vi "HEUI.vi"(0 "LED Update Rate (s)":dbl=0.25 caption="Delay Time (s)", 6 "HEUI_Buttons":T1={"SW204 - Signal Adjust"=FALSE, "SW203 - Extra Rinse"=FALSE, "SW201 - My Cycle"=FALSE, "SW202 - Delay Wash"=FALSE, "SW211 - Deep Fill"=FALSE, "SW210 - Warm Rinse"=FALSE, "SW208 - Auto Soak"=FALSE, "SW206 - Deep Rinse"=FALSE, "SW209 - Temp"=FALSE, "SW207 - Soil"=FALSE, "SW205 - Spin"=FALSE, "SW212 - Stains"=FALSE, "Cycle Selection"=enum."Cycle 0", "SW213 - Power"=FALSE, "SW214 - Start/Pause"=FALSE}, 7 "stop":bool, 11 "Error In":errorcluster) -> (5 "HEUI_LEDs":T2, 15 "Error Out":errorcluster)   [LabVIEW 2016]
doc: "This VI controls the high end 2015 VA washer UI board. The VI updates the status of the LEDs every 'LED update rate (s)' number of seconds. The VI allows the user to press buttons and select a cycle."
uses:
  Laundry Tool Support/type defs/HEUI_Buttons.ctl
  Automation/Product Specific/Clothes Care/TL27/Product Testcode/VALEW/Valew Common/Display/controls/HEUI_LEDs.ctl
  Common/LabVIEW GEA2 Toolkit/LabVIEW_GEA2_Toolkit.lvlibp/type defs/Data In.ctl
  Common/LabVIEW GEA2 Toolkit/LabVIEW_GEA2_Toolkit.lvlibp/type defs/Source_Destination.ctl
  Common/LabVIEW GEA2 Toolkit/LabVIEW_GEA2_Toolkit.lvlibp/type defs/ERD Read Data In.ctl
  Common/LabVIEW GEA2 Toolkit/LabVIEW_GEA2_Toolkit.lvlibp/type defs/Data Type.ctl
  Common/LabVIEW GEA2 Toolkit/LabVIEW_GEA2_Toolkit.lvlibp/type defs/ERD Write Data In.ctl
  Automation/Product Specific/Clothes Care/TL27/Product Testcode/VALEW/Valew Common/type defs/UI Buttons.ctl
  Common/LabVIEW GEA2 Toolkit/LabVIEW_GEA2_Toolkit.lvlibp
  Automation/Product Specific/Clothes Care/TL27/Projects/TL27.lvlib
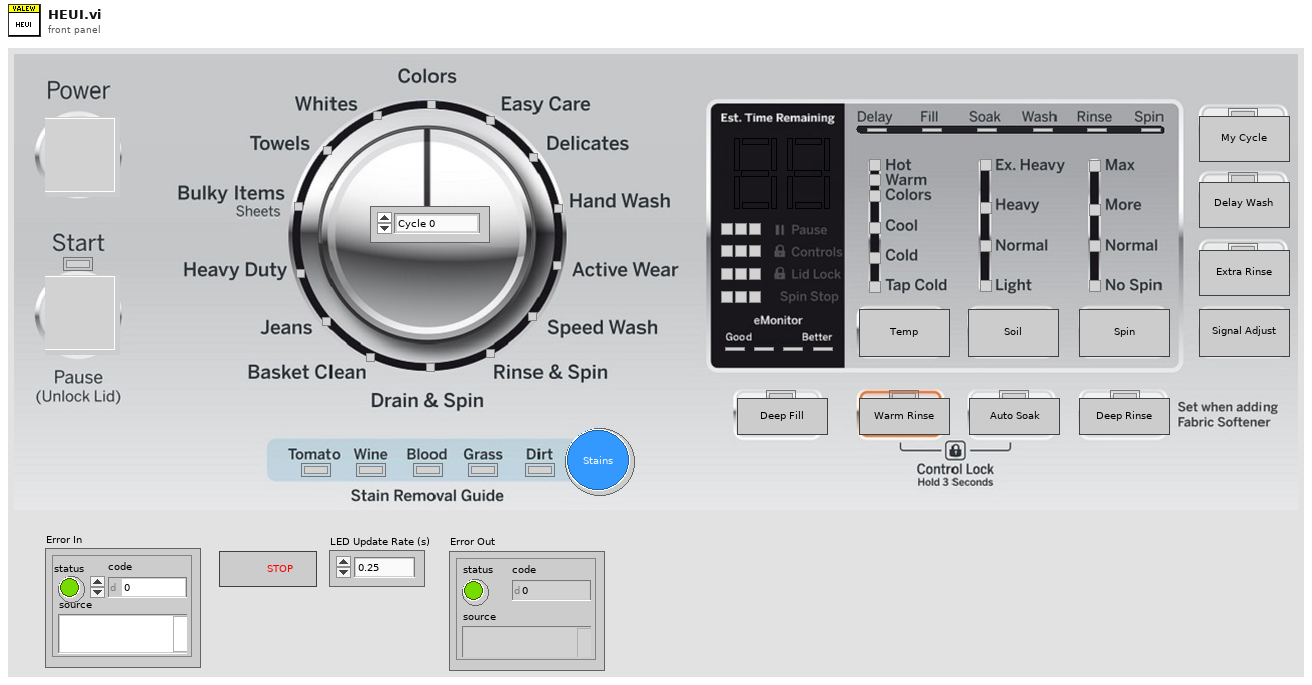
[diagram p1: front panel]
types:
  T1 = typedef "HEUI_Buttons.ctl" = cluster{"SW204 - Signal Adjust":bool, "SW203 - Extra Rinse":bool, "SW201 - My Cycle":bool, "SW202 - Delay Wash":bool, "SW211 - Deep Fill":bool, "SW210 - Warm Rinse":bool, "SW208 - Auto Soak":bool, "SW206 - Deep Rinse":bool, "SW209 - Temp":bool, "SW207 - Soil":bool, "SW205 - Spin":bool, "SW212 - Stains":bool, "Cycle Selection":enum16{"Cycle 13", "Cycle 12", "Cycle 11", "Cycle 10", "Cycle 9", "Cycle 8", "Cycle 7", "Cycle 6", "Cycle 5", "Cycle 4", "Cycle 3", "Cycle 2", "Cycle 1", "Cycle 0"}, "SW213 - Power":bool, "SW214 - Start/Pause":bool}
  T2 = typedef "TL27.lvlib/HEUI_LEDs.ctl" = cluster{"Z101 - Start":bool, "Z103 - Colors":bool, "Z104 - Whites":bool, "Z105 - Towels":bool, "Z106 - Bulky Items":bool, "Z107 - Heavy Duty":bool, "Z108 - Jeans":bool, "Z109 - Basket Clean":bool, "Z110 - Drain and Spin":bool, "Z111 - Rinse and Spin":bool, "Z112 - Speed Wash":bool, "Z113 - Active Wear":bool, "Z114 - Hand Wash":bool, "Z115 - Delicates":bool, "Z116 - Easy Care":bool, "Z117 - Tomato":bool, "Z118 - Wine":bool, "Z119 - Blood":bool, "Z120 - Grass":bool, "Z121 - Dirt":bool, "Z122_MSB_A":bool, "Z123_MSB_B":bool, "Z124_MSB_G":bool, "Z125_MSB_C":bool, "Z126_MSB_D":bool, "Z127_MSB_E":bool, "Z128_MSB_F":bool, "Z129_LSB_A":bool, "Z130_LSB_B":bool, "Z131_LSB_G":bool, "Z132_LSB_C":bool, "Z133_LSB_D":bool, "Z134_LSB_E":bool, "Z135_LSB_F":bool, "Z136 - Pause":bool, "Z137 - Pause":bool, "Z138 - Lock Controls":bool, "Z139 - Lock Controls":bool, "Z140 - Lock Controls":bool, "Z141 - Lid Lock":bool, "Z142 - Lid Lock":bool, "Z143 - Lid Lock":bool, "Z144 - Good":bool, "Z145":bool, "Z146":bool, "Z147 - Better":bool, "Z148 - Delay":bool, "Z149 - Fill":bool, "Z150 - Soak":bool, "Z151 - Wash":bool, "Z152 - Rinse":bool, "Z153 - Spin":bool, "Z154 - Hot":bool, "Z155 - Warm":bool, "Z156 - Colors":bool, "Z157 - Cool":bool, "Z158 - Cold":bool, "Z159 - Tap Cold":bool, "Z160 - Extra Heavy":bool, "Z161 - Heavy":bool, "Z162 - Normal":bool, "Z163 - Light":bool, "Z164 - Max Spin":bool, "Z165 - More Spin":bool, "Z166 - Normal Spin":bool, "Z167 - No Spin":bool, "Z168 - Extra Rinse":bool, "Z170 - Deep Rinse":bool, "Z171 - Auto Soak":bool, "Z172 - Warm Rinse":bool, "Z173 - Deep Fill":bool, "Z174 - My Cycles":bool, "Z175 - Delay Wash":bool, "Z176 - Spin Stop":bool, "Z177 - Spin Stop":bool, "Z178 - Spin Stop":bool, "Z179 - Pause":bool, "Z109":bool, "Z110":bool, "Z123":bool, "Z124":bool, "Z140":bool, "Unused0":bool, "Unused1":bool, "Unused2":bool, "Unused3":bool, "Channel_Off":bool, "Channel_Cycle_Unmapped":bool}
  T3 = typedef "LabVIEW_GEA2_Toolkit.lvlibp/ERD Write Data In.ctl" = cluster{"ERD Number":u16, "Data Type":T4, "Data":string}
  T4 = typedef "LabVIEW_GEA2_Toolkit.lvlibp/Data Type.ctl" = enum16{"string", "boolean", "uint8_t", "uint16_t", "uint32_t", "uint64_t", "int8_t", "int16_t", "int32_t", "int64_t"}
  T5 = typedef "LabVIEW_GEA2_Toolkit.lvlibp/ERD Read Data In.ctl" = cluster{"ERD Number":u16, "Data Type":T4}
  T6 = typedef "LabVIEW_GEA2_Toolkit.lvlibp/Source_Destination.ctl" = cluster{"Source":u8, "Destination":u8}
  T7 = typedef "LabVIEW_GEA2_Toolkit.lvlibp/Data In.ctl" = cluster{"Source":u8, "Destination":u8, "Command":u8, "Message":string}
  T8 = typedef "TL27.lvlib/UI Buttons.ctl" = enum16{"Switch Off", "SW201 - My Cycle", "SW202 - Delay Wash", "SW203 - Extra Rinse", "SW204 - Signal / Volume", "SW205 - Spin", "SW206 - Deep Rinse / Fab Soft", "SW207 - Soil", "SW208 - Auto Soak", "SW209 - Temp", "SW210 - Warm Rinse", "SW211 - Deep Fill", "SW212 - Stain Remover", "SW213 - Power", "SW222 - Control Lock", "SW214 - Start / Pause", "SW301 - Start/Pause LE", "SW302 - Option Button LE", "SW201/212 - Bulk Flush"}
  T9 = enum16{"string", "boolean", "uint8_t", "uint16_t", "uint32_t"}
  T10 = enum16{"Cycle 13", "Cycle 12", "Cycle 11", "Cycle 10", "Cycle 9", "Cycle 8", "Cycle 7", "Cycle 6", "Cycle 5", "Cycle 4", "Cycle 3", "Cycle 2", "Cycle 1", "Cycle 0"}
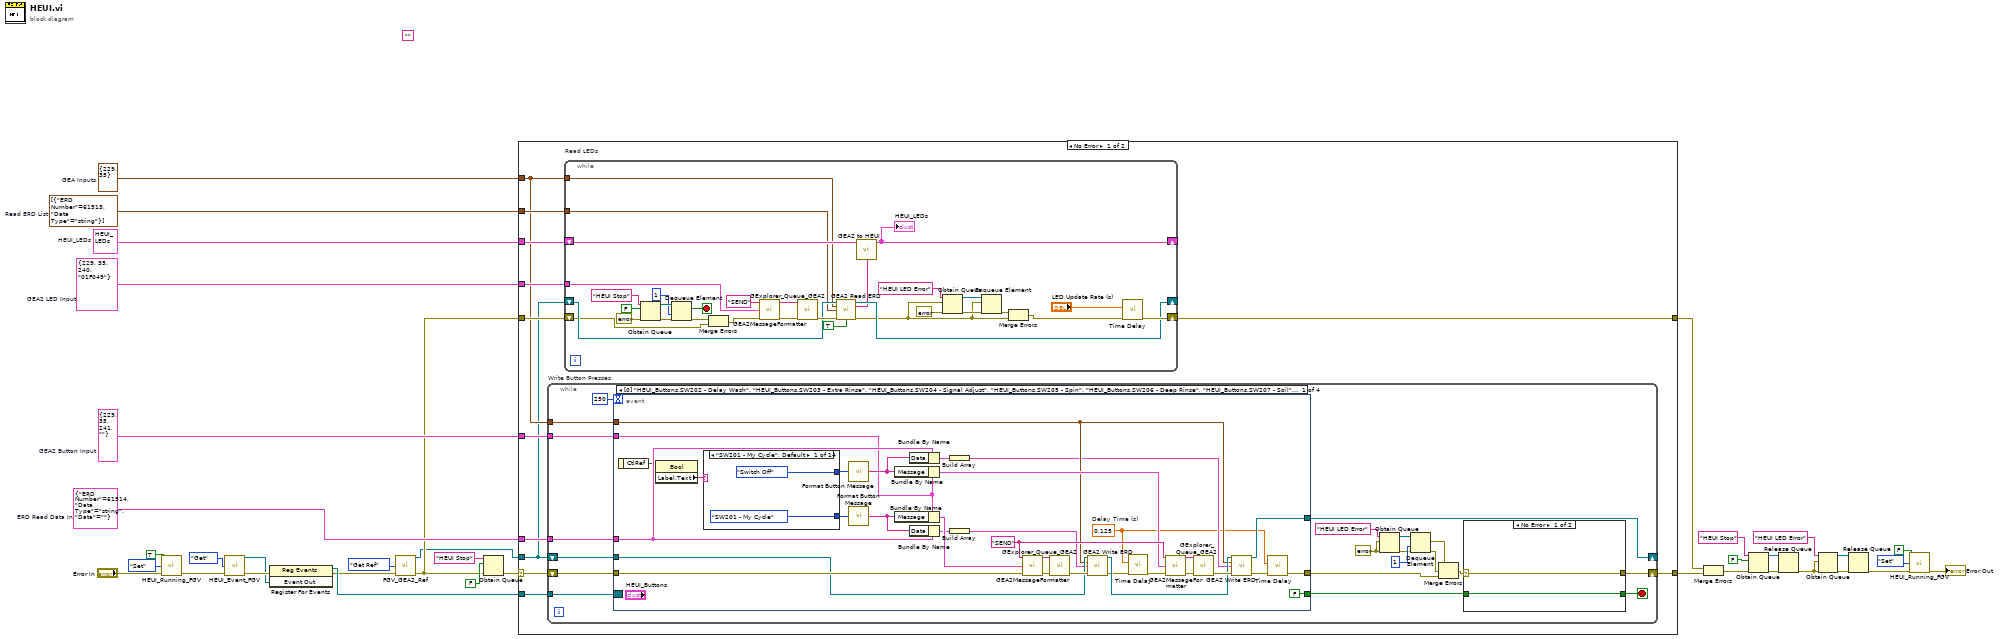
[diagram p0: block diagram]
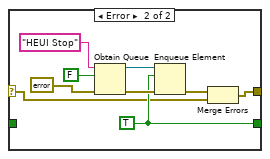
[diagram p2: hidden frame]
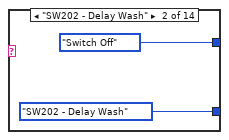
[diagram p3: hidden frame]
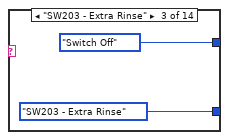
[diagram p4: hidden frame]
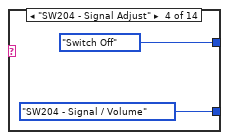
[diagram p5: hidden frame]
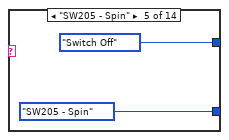
[diagram p6: hidden frame]
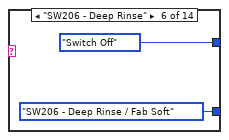
[diagram p7: hidden frame]
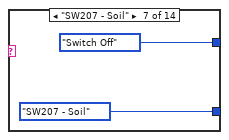
[diagram p8: hidden frame]
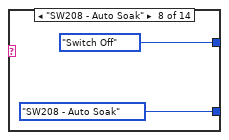
[diagram p9: hidden frame]
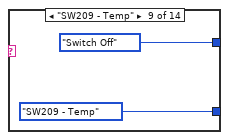
[diagram p10: hidden frame]
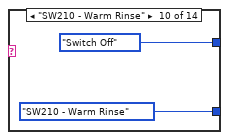
[diagram p11: hidden frame]
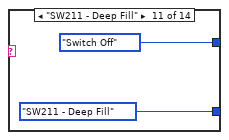
[diagram p12: hidden frame]
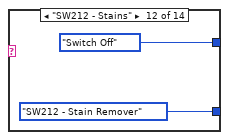
[diagram p13: hidden frame]
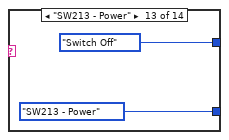
[diagram p14: hidden frame]
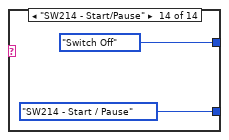
[diagram p15: hidden frame]
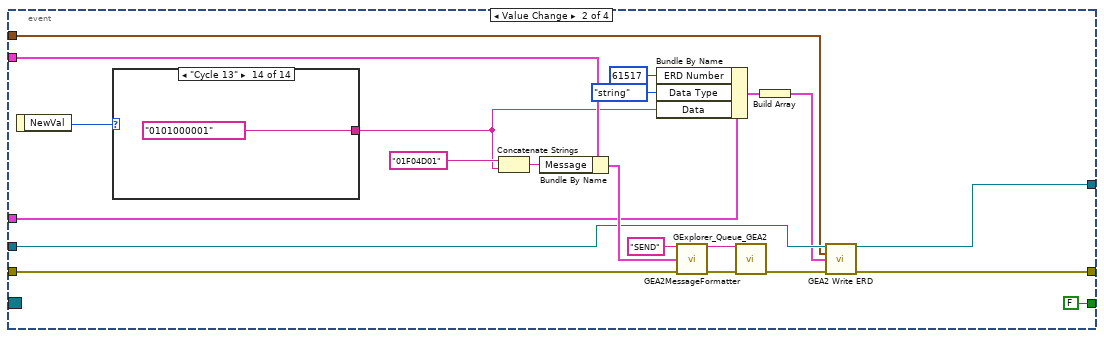
[diagram p16: hidden frame]
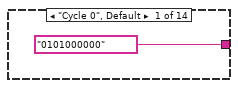
[diagram p17: hidden frame]
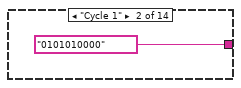
[diagram p18: hidden frame]
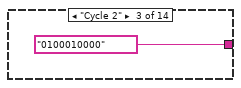
[diagram p19: hidden frame]
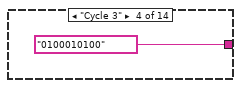
[diagram p20: hidden frame]
diagram:
  w24 = T3 {"ERD Number"=61514, "Data Type"=enum."string", "Data"=""}  # ERD Read Data In
  w26 = T5[] [{"ERD Number"=61513, "Data Type"=enum."string"}]  # Read ERD List
  w25 = T6 {"Source"=229, "Destination"=35}  # GEA Inputs
  w34 = T7 {"Source"=229, "Destination"=35, "Command"=240, "Message"="01F049"}  # GEA2 LED Input
  w35 = T2 {"Z101 - Start"=FALSE, "Z103 - Colors"=FALSE, "Z104 - Whites"=FALSE, "Z105 - Towels"=FALSE, "Z106 - Bulky Items"=FALSE, "Z107 - Heavy Duty"=FALSE, "Z108 - Jeans"=FALSE, "Z109 - Basket Clean"=FALSE, "Z110 - Drain and Spin"=FALSE, "Z111 - Rinse and Spin"=FALSE, "Z112 - Speed Wash"=FALSE, "Z113 - Active Wear"=FALSE, "Z114 - Hand Wash"=FALSE, "Z115 - Delicates"=FALSE, "Z116 - Easy Care"=FALSE, "Z117 - Tomato"=FALSE, "Z118 - Wine"=FALSE, "Z119 - Blood"=FALSE, "Z120 - Grass"=FALSE, "Z121 - Dirt"=FALSE, "Z122_MSB_A"=FALSE, "Z123_MSB_B"=FALSE, "Z124_MSB_G"=FALSE, "Z125_MSB_C"=FALSE, "Z126_MSB_D"=FALSE, "Z127_MSB_E"=FALSE, "Z128_MSB_F"=FALSE, "Z129_LSB_A"=FALSE, "Z130_LSB_B"=FALSE, "Z131_LSB_G"=FALSE, "Z132_LSB_C"=FALSE, "Z133_LSB_D"=FALSE, "Z134_LSB_E"=FALSE, "Z135_LSB_F"=FALSE, "Z136 - Pause"=FALSE, "Z137 - Pause"=FALSE, "Z138 - Lock Controls"=FALSE, "Z139 - Lock Controls"=FALSE, "Z140 - Lock Controls"=FALSE, "Z141 - Lid Lock"=FALSE, "Z142 - Lid Lock"=FALSE, "Z143 - Lid Lock"=FALSE, "Z144 - Good"=FALSE, "Z145"=FALSE, "Z146"=FALSE, "Z147 - Better"=FALSE, "Z148 - Delay"=FALSE, "Z149 - Fill"=FALSE, "Z150 - Soak"=FALSE, "Z151 - Wash"=FALSE, "Z152 - Rinse"=FALSE, "Z153 - Spin"=FALSE, "Z154 - Hot"=FALSE, "Z155 - Warm"=FALSE, "Z156 - Colors"=FALSE, "Z157 - Cool"=FALSE, "Z158 - Cold"=FALSE, "Z159 - Tap Cold"=FALSE, "Z160 - Extra Heavy"=FALSE, "Z161 - Heavy"=FALSE, "Z162 - Normal"=FALSE, "Z163 - Light"=FALSE, "Z164 - Max Spin"=FALSE, "Z165 - More Spin"=FALSE, "Z166 - Normal Spin"=FALSE, "Z167 - No Spin"=FALSE, "Z168 - Extra Rinse"=FALSE, "Z170 - Deep Rinse"=FALSE, "Z171 - Auto Soak"=FALSE, "Z172 - Warm Rinse"=FALSE, "Z173 - Deep Fill"=FALSE, "Z174 - My Cycles"=FALSE, "Z175 - Delay Wash"=FALSE, "Z176 - Spin Stop"=FALSE, "Z177 - Spin Stop"=FALSE, "Z178 - Spin Stop"=FALSE, "Z179 - Pause"=FALSE, "Z109"=FALSE, "Z110"=FALSE, "Z123"=FALSE, "Z124"=FALSE, "Z140"=FALSE, "Unused0"=FALSE, "Unused1"=FALSE, "Unused2"=FALSE, "Unused3"=FALSE, "Channel_Off"=FALSE, "Channel_Cycle_Unmapped"=FALSE}  # HEUI_LEDs
  w33 = T7 {"Source"=229, "Destination"=35, "Command"=241, "Message"=""}  # GEA2 Button Input
  (unwired) ""
  n1 = call "HEUI_Running_FGV.vi"("Running?"=TRUE, "Action"=enum16{"Get", "Set"}."Set", "Error In"="Error In") -> ("Error Out"=w8:errorcluster)  [unwired: 11 in, 1 out]
  n2 = call "HEUI_Event_FGV.vi"("Action"=enum16{"Get", "Set"}."Get", "Error In"=w8) -> ("Event Out"=w15:refnum<user-event>, "Error Out"=w16:errorcluster)  [unwired: 12 in]
  n3 = register-events(error in=w16, w15) -> (reference out=w18:refnum<event-registration>, error out=w12:errorcluster)  [unwired: 1 in]
  n4 = call "FGV_GEA2_Ref.vi"("Action"=enum16{"Set Ref", "Get Ref"}."Get Ref", "Error In"=w12) -> ("GEA2 Reference Out"=w10:refnum<k24>, "Error Out"=w11:errorcluster)  [unwired: 12 in]
  n5 = Obtain Queue(name (unnamed)="HEUI Stop", element data type=FALSE ("stop"), error in (no error)=w11) -> (error out=w23:errorcluster)  [unwired: 2 in, 2 out]
  n6 = case shown="No Error" w23 {
    selector: w23 -> [w38 w238]
    tunnel: w10 -> [w39 _]
    tunnel: [w48 errorcluster {"status"=FALSE, "code"=0, "source"=""} ("error out")] -> w36
    tunnel: [w47 w238] -> w9
    tunnel: w35 -> [w46 _]
    tunnel: w34 -> [w45 _]
    tunnel: w33 -> [w44 _]
    tunnel: w11 -> [w43 _]
    tunnel: w26 -> [w42 _]
    tunnel: w25 -> [w41 _]
    tunnel: w24 -> [w40 _]
    tunnel: w18 -> [w37 _]
    frame No Error {
      n7 = while "Write Button Presses" {
        shift-right: [w94] -> w47
        shift-left: w38 -> [w100]
        shift-right: [w98] -> _
        shift-left: w39 -> [w99]
        tunnel: w44 -> [w97]
        tunnel: w41 -> [w96]
        tunnel: w40 -> [w95]
        tunnel: w37 -> [w81]
        stop <- w92 stop-if-true
        w86 = errorcluster {"status"=FALSE, "code"=0, "source"=""} ("error in (no error)")
        n8 = event shown="[0] \"HEUI_Buttons.SW202 - Delay Wash\", \"HEUI_Buttons.SW203 - Extra Rinse\", \"HEUI_Buttons.SW204 - Signal Adjust\", \"HEUI_Buttons.SW205 - Spin\", \"HEUI_Buttons.SW206 - Deep Rinse\", \"HEUI_Buttons.SW207 - Soil\", \"HEUI_Buttons.SW208 - Auto Soak\", \"HEUI_Buttons.SW209 - Temp\", \"HEUI_Buttons.SW210 - Warm Rinse\", \"HEUI_Buttons.SW211 - Deep Fill\", \"HEUI_Buttons.SW212 - Stains\", \"HEUI_Buttons.SW213 - Power\", \"HEUI_Buttons.SW214 - Start/Pause\", \"HEUI_Buttons.SW201 - My Cycle\": Value Change" {
          selector: w81 -> [_ _ _ _]
          dyn-events: _ -> [_ _ _ _]
          timeout: 250 -> [_ _ _ _]
          tunnel: [w120 w184 w232 w235] -> w84
          tunnel: w100 -> [w142 w192 w213 w235]
          tunnel: w99 -> [w134 w183 w209 w236]
          tunnel: [w132 w182 w207 w236] -> w98
          tunnel: [FALSE ("stop") FALSE ("stop") w231 FALSE ("stop")] -> w93
          tunnel: w97 -> [w117 w191 w215 _]
          tunnel: w96 -> [w130 w181 w208 _]
          tunnel: w95 -> [w125 w180 w211 _]
          event Value Change {
            w116 = 0.125  # Delay Time (s)
            w140 = "SEND" ("Prefix(Send/Recv)")
            n9 = event-data() -> ("CtlRef"=w119:refnum<vi>)  [unwired: 1 in]
            n10 = property class="Bool"(reference=w119) -> ("Label.Text"=w118:string)  [unwired: 1 in, 2 out]
            n11 = case shown="\"SW201 - My Cycle\", Default" w118 {
              tunnel: [UI_Buttons."SW201 - My Cycle" ("Switch") UI_Buttons."SW202 - Delay Wash" ("Switch") UI_Buttons."SW203 - Extra Rinse" ("Switch") UI_Buttons."SW204 - Signal / Volume" ("Switch") UI_Buttons."SW205 - Spin" ("Switch") UI_Buttons."SW206 - Deep Rinse / Fab Soft" ("Switch") UI_Buttons."SW207 - Soil" ("Switch") UI_Buttons."SW208 - Auto Soak" ("Switch") UI_Buttons."SW209 - Temp" ("Switch") UI_Buttons."SW210 - Warm Rinse" ("Switch") UI_Buttons."SW211 - Deep Fill" ("Switch") UI_Buttons."SW212 - Stain Remover" ("Switch") UI_Buttons."SW213 - Power" ("Switch") UI_Buttons."SW214 - Start / Pause" ("Switch")] -> w113
              tunnel: [UI_Buttons."Switch Off" ("Switch") UI_Buttons."Switch Off" ("Switch") UI_Buttons."Switch Off" ("Switch") UI_Buttons."Switch Off" ("Switch") UI_Buttons."Switch Off" ("Switch") UI_Buttons."Switch Off" ("Switch") UI_Buttons."Switch Off" ("Switch") UI_Buttons."Switch Off" ("Switch") UI_Buttons."Switch Off" ("Switch") UI_Buttons."Switch Off" ("Switch") UI_Buttons."Switch Off" ("Switch") UI_Buttons."Switch Off" ("Switch") UI_Buttons."Switch Off" ("Switch") UI_Buttons."Switch Off" ("Switch")] -> w114
              frame "SW201 - My Cycle", Default {
              }
              frame "SW202 - Delay Wash" {
              }
              frame "SW203 - Extra Rinse" {
              }
              frame "SW204 - Signal Adjust" {
              }
              frame "SW205 - Spin" {
              }
              frame "SW206 - Deep Rinse" {
              }
              frame "SW207 - Soil" {
              }
              frame "SW208 - Auto Soak" {
              }
              frame "SW209 - Temp" {
              }
              frame "SW210 - Warm Rinse" {
              }
              frame "SW211 - Deep Fill" {
              }
              frame "SW212 - Stains" {
              }
              frame "SW213 - Power" {
              }
              frame "SW214 - Start/Pause" {
              }
            }
            n12 = call "Format Button Message.vi"("Switch"=w114) -> ("Switch Message"=w129:string)  [unwired: 14 in]
            n13 = call "Format Button Message.vi"("Switch"=w113) -> ("Switch Message"=w112:string)  [unwired: 14 in]
            n14 = Bundle By Name(cluster=w117, "Message"=w129) -> (w136:T7)
            n15 = Bundle By Name(cluster=w117, "Message"=w112) -> (w137:T7)
            n16 = Bundle By Name(cluster=w125, "Data"=w129) -> (w128:T3)
            n17 = Bundle By Name(cluster=w125, "Data"=w112) -> (w126:T3)
            n18 = Build Array(w128) -> (w127:T3[])
            n19 = Build Array(w126) -> (w124:T3[])
            n20 = call "GEA2MessageFormatter.vi"("Prefix(Send/Recv)"=w140, "GEA2 Data In"=w137, "Error In"=w142) -> ("Output String"=w139:string, "Error Out"=w143:errorcluster)  [unwired: 11 in]
            n21 = call "GExplorer_Queue_GEA2.vi"("Output String"=w139, "error in (no error)"=w143) -> ("error out"=w135:errorcluster)  [unwired: 13 in]
            n22 = call "GEA2 Write ERD.vi"("GEA2 Reference In"=w134, "GEA Inputs"=w130, "Write ERD List"=w124, "Error In"=w135) -> ("GEA2 Reference Out"=w131:refnum<k24>, "Error Out"=w123:errorcluster)  [unwired: 9 in, 1 out]
            n23 = call "Time Delay"("error in (no error)"=w123, "Delay Time (s)"=w116) -> ("error out"=w122:errorcluster)  [unwired: 9 in]
            n24 = call "GEA2MessageFormatter.vi"("Prefix(Send/Recv)"=w140, "GEA2 Data In"=w136, "Error In"=w122) -> ("Output String"=w138:string, "Error Out"=w141:errorcluster)  [unwired: 11 in]
            n25 = call "GExplorer_Queue_GEA2.vi"("Output String"=w138, "error in (no error)"=w141) -> ("error out"=w133:errorcluster)  [unwired: 13 in]
            n26 = call "GEA2 Write ERD.vi"("GEA2 Reference In"=w131, "GEA Inputs"=w130, "Write ERD List"=w127, "Error In"=w133) -> ("GEA2 Reference Out"=w132:refnum<k24>, "Error Out"=w121:errorcluster)  [unwired: 9 in, 1 out]
            n27 = call "Time Delay"("error in (no error)"=w121, "Delay Time (s)"=w116) -> ("error out"=w120:errorcluster)  [unwired: 9 in]
          }
          event Value Change {
            n28 = event-data() -> ("NewVal"=w175:T10)  [unwired: 1 in]
            n29 = case shown="\"Cycle 13\"" w175 {
              tunnel: ["0101000000" "0101010000" "0100010000" "0100010100" "0101010100" "0101000100" "0100000100" "0100000101" "0101000101" "0101010101" "0100010101" "0100010001" "0101010001" "0101000001"] -> w173
              frame "Cycle 0", Default {
              }
              frame "Cycle 1" {
              }
              frame "Cycle 2" {
              }
              frame "Cycle 3" {
              }
              frame "Cycle 4" {
              }
              frame "Cycle 5" {
              }
              frame "Cycle 6" {
              }
              frame "Cycle 7" {
              }
              frame "Cycle 8" {
              }
              frame "Cycle 9" {
              }
              frame "Cycle 10" {
              }
              frame "Cycle 11" {
              }
              frame "Cycle 12" {
              }
              frame "Cycle 13" {
              }
            }
            n30 = Concatenate Strings("01F04D01" ("string"), w173) -> (w174:string)
            n31 = Bundle By Name(cluster=w191, "Message"=w174) -> (w187:T7)
            n32 = Bundle By Name(cluster=w180, "ERD Number"=u16 61517, "Data Type"=T9."string", "Data"=w173) -> (w177:T3)
            n33 = call "GEA2MessageFormatter.vi"("Prefix(Send/Recv)"="SEND", "GEA2 Data In"=w187, "Error In"=w192) -> ("Output String"=w186:string, "Error Out"=w190:errorcluster)  [unwired: 11 in]
            n34 = call "GExplorer_Queue_GEA2.vi"("Output String"=w186, "error in (no error)"=w190) -> ("error out"=w185:errorcluster)  [unwired: 13 in]
            n35 = Build Array(w177) -> (w176:T3[])
            n36 = call "GEA2 Write ERD.vi"("GEA2 Reference In"=w183, "GEA Inputs"=w181, "Write ERD List"=w176, "Error In"=w185) -> ("GEA2 Reference Out"=w182:refnum<k24>, "Error Out"=w184:errorcluster)  [unwired: 9 in, 1 out]
          }
          event "stop": Value Change; Panel Close; User Event {
            w214 = "0000000000" ("string")
            w231 = TRUE ("stop")
            n37 = event-data() -> ()  [unwired: 1 in, 1 out]
            n38 = Concatenate Strings("01F04D01" ("string"), w214) -> (w216:string)
            n39 = Bundle By Name(cluster=w215, "Message"=w216) -> (w222:T7)
            n40 = Bundle By Name(cluster=w211, "ERD Number"=u16 61517, "Data Type"=T9."string", "Data"=w214) -> (w217:T3)
            n41 = call "GEA2MessageFormatter.vi"("Prefix(Send/Recv)"="SEND", "GEA2 Data In"=w222, "Error In"=w213) -> ("Output String"=w221:string, "Error Out"=w225:errorcluster)  [unwired: 11 in]
            n42 = call "GExplorer_Queue_GEA2.vi"("Output String"=w221, "error in (no error)"=w225) -> ("error out"=w220:errorcluster)  [unwired: 13 in]
            n43 = Build Array(w217) -> (w210:T3[])
            n44 = call "GEA2 Write ERD.vi"("GEA2 Reference In"=w209, "GEA Inputs"=w208, "Write ERD List"=w210, "Error In"=w220) -> ("GEA2 Reference Out"=w207:refnum<k24>, "Error Out"=w212:errorcluster)  [unwired: 9 in, 1 out]
            n45 = control-ref of="This VI"() -> (w233:refnum<vi>)
            n46 = invoke class="VI" method="FP.Close"(reference=w233, error in=w212) -> (error out=w230:errorcluster)  [unwired: 1 in, 2 out]
            n47 = Obtain Queue(name (unnamed)="HEUI Stop", element data type=FALSE ("stop"), error in (no error)=w230) -> (queue out=w228:refnum<queue>, error out=w229:errorcluster)  [unwired: 2 in, 1 out]
            n48 = Enqueue Element(queue=w228, element=w231, error in (no error)=w229) -> (error out=w232:errorcluster)  [unwired: 1 in, 2 out]
          }
          event Timeout {
            n49 = event-data() -> ()  [unwired: 1 in, 3 out]
          }
        }
        n50 = Obtain Queue(name (unnamed)="HEUI LED Error", element data type=w86, error in (no error)=w86) -> (queue out=w88:refnum<queue>, error out=w89:errorcluster)  [unwired: 2 in, 1 out]
        n51 = Dequeue Element(queue=w88, timeout in ms (-1)=1, error in (no error)=w89) -> (element=w82:errorcluster, error out=w83:errorcluster)  [unwired: 2 out]
        n52 = Merge Errors(w82, w83, w84) -> (w87:errorcluster)
        n53 = case shown="No Error" w87 {
          selector: w87 -> [w102 w104]
          tunnel: [w102 w106] -> w94
          tunnel: w93 -> [w101 _]
          tunnel: [w101 w107] -> w92
          frame No Error {
          }
          frame Error {
            w107 = TRUE ("stop")
            n54 = Obtain Queue(name (unnamed)="HEUI Stop", element data type=FALSE ("stop"), error in (no error)=errorcluster {"status"=FALSE, "code"=0, "source"=""}) -> (queue out=w110:refnum<queue>, error out=w111:errorcluster)  [unwired: 2 in, 1 out]
            n55 = Enqueue Element(queue=w110, element=w107, error in (no error)=w111) -> (error out=w105:errorcluster)  [unwired: 1 in, 2 out]
            n56 = Merge Errors(w105, w104) -> (w106:errorcluster)
          }
        }
      }
      n57 = while "Read LEDs" {
        shift-right: [w78] -> w48
        shift-left: w43 -> [w49]
        shift-right: [w65] -> _
        shift-left: w39 -> [w64]
        tunnel: w45 -> [w73]
        tunnel: w41 -> [w63]
        tunnel: w42 -> [w62]
        shift-right: [w80] -> _
        shift-left: w46 -> [w79]
        stop <- w72 stop-if-true
        n58 = Obtain Queue(name (unnamed)="HEUI Stop", element data type=FALSE ("stop"), error in (no error)=errorcluster {"status"=FALSE, "code"=0, "source"=""}) -> (queue out=w71:refnum<queue>, error out=w70:errorcluster)  [unwired: 2 in, 1 out]
        n59 = Dequeue Element(queue=w71, timeout in ms (-1)=1, error in (no error)=w70) -> (element=w72:bool, error out=w52:errorcluster)  [unwired: 2 out]
        n60 = Merge Errors(w52, w49) -> (w51:errorcluster)
        n61 = call "GEA2MessageFormatter.vi"("Prefix(Send/Recv)"="SEND", "GEA2 Data In"=w73, "Error In"=w51) -> ("Output String"=w75:string, "Error Out"=w74:errorcluster)  [unwired: 11 in]
        n62 = call "GExplorer_Queue_GEA2.vi"("Output String"=w75, "error in (no error)"=w74) -> ("error out"=w66:errorcluster)  [unwired: 13 in]
        n63 = call "GEA2 Read ERD.vi"("GEA2 Reference In"=w64, "GEA Inputs"=w63, "Read ERD List"=w62, "Error In"=w66, "Verify ERD Response?"=TRUE) -> ("GEA2 Reference Out"=w65:refnum<k24>, "Raw Data Out"=w61:string, "Error Out"=w55:errorcluster)  [unwired: 7 in, 1 out]
        n64 = call "GEA2 to HEUI.vi"("HEUI_LEDs_In"=w79, "Raw Data In"=w61) -> ("HEUI_LEDs_Out"=w80:T2)  [unwired: 13 in]
        "HEUI_LEDs" <- w80
        n65 = Obtain Queue(name (unnamed)="HEUI LED Error", element data type=w55, error in (no error)=errorcluster {"status"=FALSE, "code"=0, "source"=""}) -> (queue out=w58:refnum<queue>, error out=w57:errorcluster)  [unwired: 2 in, 1 out]
        n66 = Enqueue Element(queue=w58, element=w55, error in (no error)=w57) -> (error out=w56:errorcluster)  [unwired: 1 in, 2 out]
        n67 = Merge Errors(w56, w55) -> (w54:errorcluster)
        n68 = call "Time Delay"("error in (no error)"=w54, "Delay Time (s)"="LED Update Rate (s)") -> ("error out"=w78:errorcluster)  [unwired: 9 in]
      }
    }
    frame Error {
    }
  }
  n69 = Merge Errors(w36, w9) -> (w14:errorcluster)
  n70 = Obtain Queue(name (unnamed)="HEUI Stop", element data type=FALSE ("stop"), error in (no error)=w14) -> (queue out=w27:refnum<queue>, error out=w28:errorcluster)  [unwired: 2 in, 1 out]
  n71 = Release Queue(queue=w27, error in (no error)=w28) -> (error out=w19:errorcluster)  [unwired: 1 in, 2 out]
  n72 = Obtain Queue(name (unnamed)="HEUI LED Error", element data type=w19, error in (no error)=w19) -> (queue out=w22:refnum<queue>, error out=w21:errorcluster)  [unwired: 2 in, 1 out]
  n73 = Release Queue(queue=w22, error in (no error)=w21) -> (error out=w3:errorcluster)  [unwired: 1 in, 2 out]
  n74 = call "HEUI_Running_FGV.vi"("Running?"=FALSE, "Action"=enum16{"Get", "Set"}."Set", "Error In"=w3) -> ("Error Out"=→"Error Out":errorcluster)  [unwired: 11 in, 1 out]
